vi "Data flow.vi"(0 "x":dbl=1.0 format="%.2f", 1 "y":dbl format="%.2f") -> (2 "x+y":dbl format="%.2f", 3 "Molt-somma":dbl, 4 "Somma-molt":dbl, 5 "2*x":dbl format="%.2f")   [LabVIEW 2012]
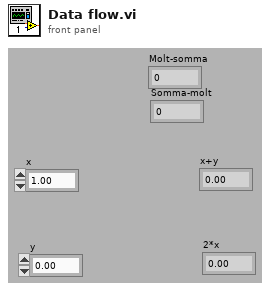
[diagram p1: front panel]
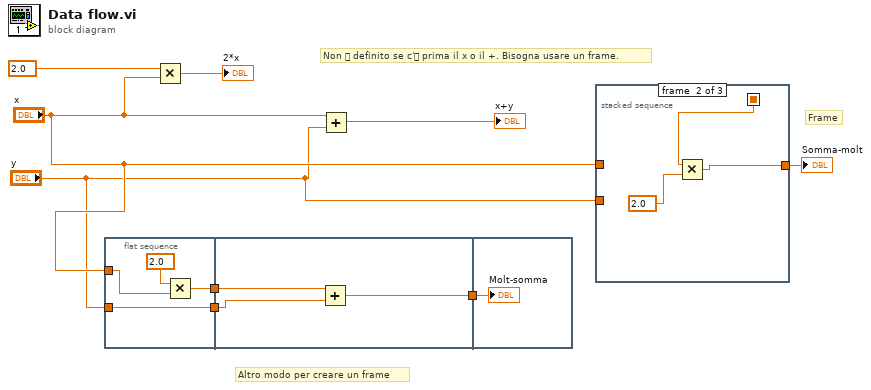
[diagram p0: block diagram]
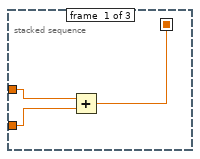
[diagram p2: hidden frame]
diagram:
  # "Non  definito se c' prima il x o il +. Bisogna usare un frame."
  # "Frame"
  # "Altro modo per creare un frame"
  n1 = flat-sequence {
    tunnel: "x" -> [w12]
    tunnel: "y" -> [w13]
    tunnel: [w13] -> w4
    tunnel: [w10] -> w3
    tunnel: w4 -> [w15]
    tunnel: w3 -> [w16]
    tunnel: [w14] -> w2
    tunnel: w2 -> [w17]
    frame #0 {
      n2 = Multiply(x=2.0 ("y"), y=w12) -> (x*y=w10:dbl)
    }
    frame #1 {
      n3 = Add(x=w16, y=w15) -> (x+y=w14:dbl)
    }
    frame #2 {
      "Molt-somma" <- w17
    }
  }
  n4 = Multiply(x=2.0 ("y"), y="x") -> (x*y=→"2*x":dbl)
  n5 = Add(x="x", y="y") -> (x+y=→"x+y":dbl)
  n6 = stacked-sequence {
    seq-local: [w18 _ _] -> [_ w22 _]
    tunnel: "x" -> [w20 _ _]
    tunnel: "y" -> [w19 _ _]
    tunnel: [_ w21 _] -> w1
    frame #0 {
      n7 = Add(x=w20, y=w19) -> (x+y=w18:dbl)
    }
    frame #1 {
      n8 = Multiply(x=w22, y=2.0) -> (x*y=w21:dbl)
    }
    frame #2 {
    }
  }
  "Somma-molt" <- w1
